vi "GoalFound.vi"(11 "Start Goal Data":T1) -> (3 "Start Goal Data out":T1, 5 "Boolean":bool)   [LabVIEW 2013]
uses:
  Bug_StartGoalData.ctl
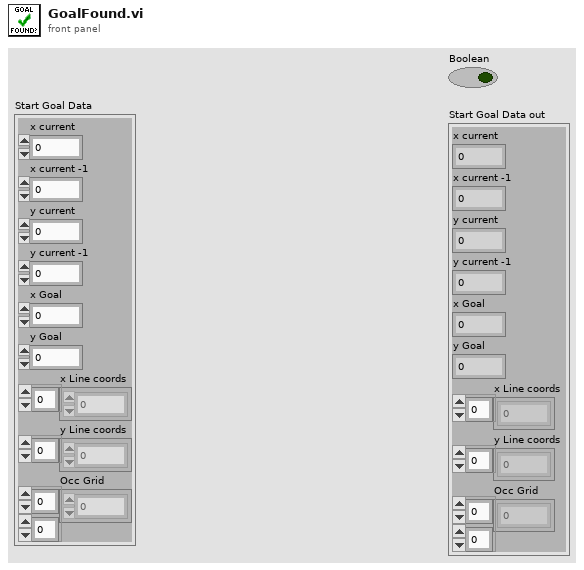
[diagram p1: front panel]
types:
  T1 = typedef "Bug_StartGoalData.ctl" = cluster{"x current":i32, "x current -1":i32, "y current":i32, "y current -1":i32, "x Goal":i32, "y Goal":i32, "x Line coords":i32[], "y Line coords":i32[], "Occ Grid":dbl[][]}
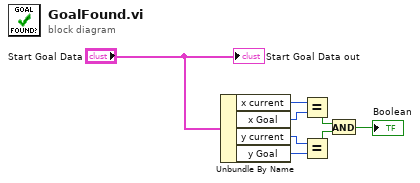
[diagram p0: block diagram]
diagram:
  n1 = Unbundle By Name("Start Goal Data") -> ("x current"=w8:i32, "x Goal"=w6:i32, "y current"=w5:i32, "y Goal"=w7:i32)
  n2 = Equal?(x=w8, y=w6) -> (x = y?=w3:bool)
  n3 = Equal?(x=w5, y=w7) -> (x = y?=w4:bool)
  n4 = And(x=w3, y=w4) -> (x .and. y?=→"Boolean":bool)
  "Start Goal Data out" <- "Start Goal Data"
